vi "Sandbox 3.vi"() -> ()   [LabVIEW 2020]
panel:
  out "error out 2":errorcluster
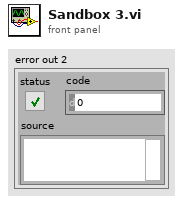
[diagram p1: front panel]
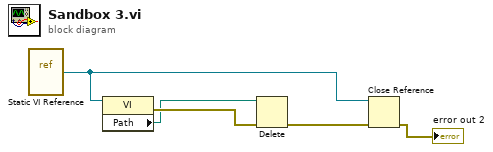
[diagram p0: block diagram]
diagram:
  n1 = vi-ref "Static VI Reference"() -> ("vi reference"=w1:refnum<vi>)
  n2 = property class="VI"(reference=w1) -> (error out=w4:errorcluster, "Path"=w3:path)  [unwired: 1 in, 1 out]
  n3 = Delete(path (use dialog)=w3, error in=w4) -> (error out=w2:errorcluster)  [unwired: 3 in, 2 out]
  n4 = Close Reference(reference=w1, error in (no error)=w2) -> (error out=→"error out 2":errorcluster)
